vi "Tab Control - Change to TabName Heatup.vi"(0 "TabCtl Refnum":refnum<vi>, 1 "Label.Text":string) -> ()   [LabVIEW 2013]
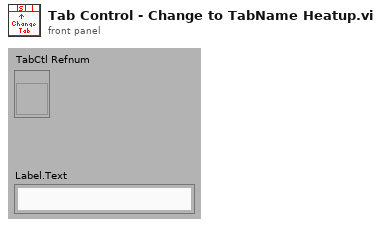
[diagram p1: front panel]
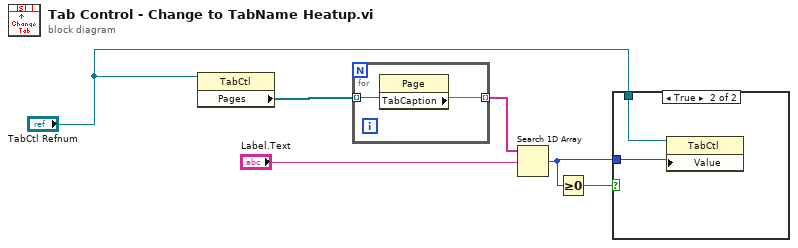
[diagram p0: block diagram]
diagram:
  n1 = property class="TabCtl"(reference="TabCtl Refnum") -> ("Pages"=w6:refnum<vi>[])  [unwired: 1 in, 2 out]
  n2 = for {
    tunnel: w6 -> [w7] mode=indexing
    tunnel: [w8] -> w5 mode=indexing
    n3 = property class="Page"(reference=w7) -> ("TabCaption"=w8:string)  [unwired: 1 in, 2 out]
  }
  n4 = Search 1D Array(1D array=w5, element="Label.Text") -> (index of element=w2:i32)  [unwired: 1 in]
  n5 = Greater Or Equal To 0?(x=w2) -> (x >= 0?=w3:bool)
  n6 = case shown="True" w3 {
    tunnel: w2 -> [_ w10]
    tunnel: "TabCtl Refnum" -> [_ w9]
    frame False {
    }
    frame True {
      n7 = property class="TabCtl"(reference=w9, "Value"=w10) -> ()  [unwired: 1 in, 2 out]
    }
  }
